vi "SmartDelay.vi"(11 "Frequency":dbl) -> ()   [LabVIEW 2014]
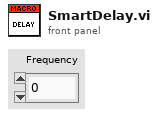
[diagram p1: front panel]
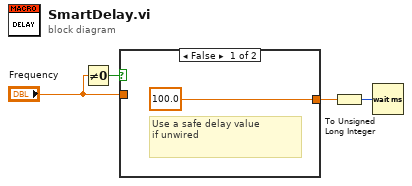
[diagram p0: block diagram]
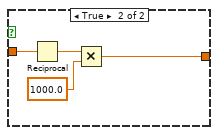
[diagram p2: hidden frame]
diagram:
  n1 = Not Equal To 0?(x="Frequency") -> (x != 0?=w4:bool)
  n2 = case shown="False" w4 {
    tunnel: "Frequency" -> [_ w7]
    tunnel: [100.0 w6] -> w2
    frame False {
      # "Use a safe delay value\nif unwired"
    }
    frame True {
      n3 = Reciprocal(x=w7) -> (1/x=w9:dbl)
      n4 = Multiply(x=w9, y=1000.0) -> (x*y=w6:dbl)
    }
  }
  n5 = To Unsigned Long Integer(number=w2) -> (unsigned 32bit integer=w1:u32)
  n6 = Wait (ms)(milliseconds to wait=w1) -> ()  [unwired: 1 out]
